vi "GetParam.vi"(8 "error in (no error)":errorcluster caption="entrée d'erreur (pas d'erreur)", 11 "Covtype.lvclass":refnum<class "Covtype.lvclass">) -> (0 "error out":errorcluster caption="sortie d'erreur", 2 "fetch_covtype":T1={"download_if_missing"=TRUE, "random_state"=-1, "shuffle"=TRUE, "Returns"="Data"} {"random_state" min=-1}, 3 "Covtype.lvclass":refnum<class "Covtype.lvclass">)   [LabVIEW 2020, in "Covtype.lvclass"]
doc: "Get parameters"
uses:
  Covtype.lvclass
  Covtype.lvclass/Covtype.ctl
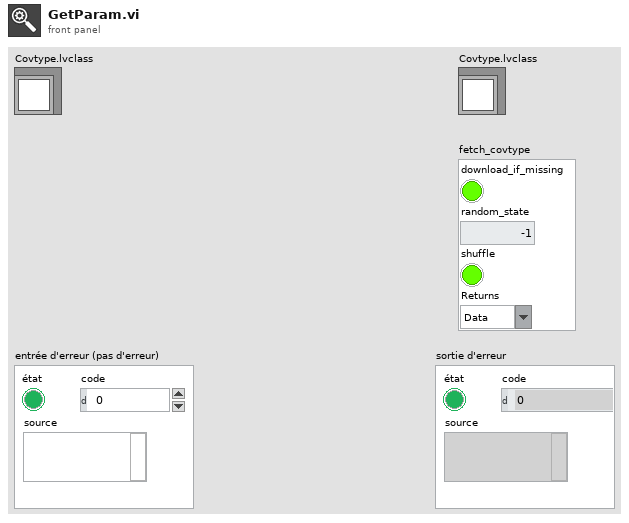
[diagram p1: front panel]
types:
  T1 = cluster{"download_if_missing":bool, "random_state":i32, "shuffle":bool, "Returns":string}
  T2 = cluster{" download_if_missing ":bool, "random_state":i32, "shuffle":bool, "Returns":string}
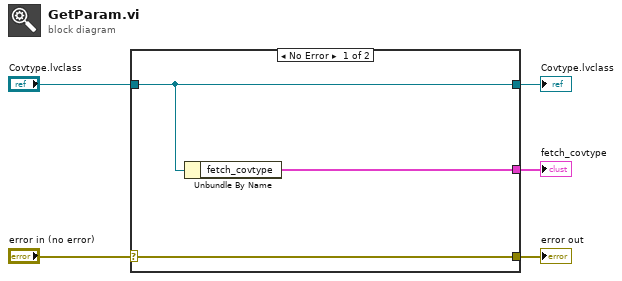
[diagram p0: block diagram]
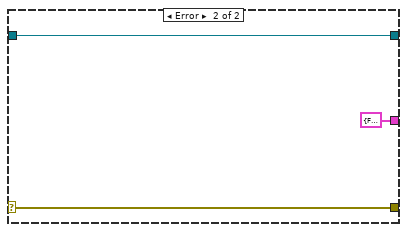
[diagram p2: hidden frame]
diagram:
  n1 = case shown="No Error" "error in (no error)" {
    selector: "error in (no error)" -> [w8 w10]
    tunnel: [w8 w10] -> w4
    tunnel: [w7 w11] -> w2
    tunnel: "Covtype.lvclass" -> [w7 w11]
    tunnel: [w6 T2 {" download_if_missing "=FALSE, "random_state"=0, "shuffle"=FALSE, "Returns"=""} ("fetch_covtype")] -> w1
    frame No Error {
      n2 = Unbundle By Name(w7) -> ("fetch_covtype"=w6:T2)
    }
    frame Error {
    }
  }
  "error out" <- w4
  "Covtype.lvclass" <- w2
  "fetch_covtype" <- w1
